vi "file - read list of lines.vi"(11 "file path":path=path "\\\\rus-one\\newdata/data/Ultrasound/Experiment/ProbeTest/Probe10/Hg1201-6-C185-550Cair-3c-83K/sweep3/9w/3366_a.dat") -> (1 "first line":string, 2 "list of lines":string[](array[string]))   [LabVIEW 2015]
uses:
  <vilib>/Utility/file.llb/Read From Spreadsheet File (string).vi
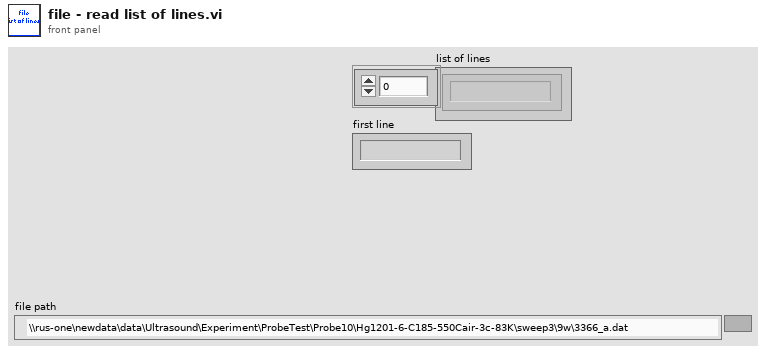
[diagram p1: front panel]
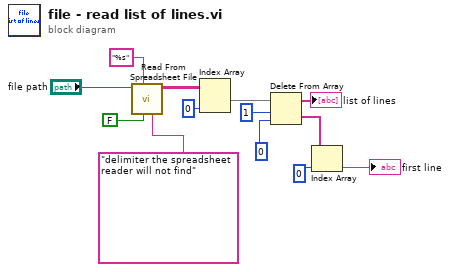
[diagram p0: block diagram]
diagram:
  n1 = call-poly <vilib>:"Read From Spreadsheet File.vi"("delimiter (\\t)"="delimiter the spreadsheet reader will not find" ("delimiter (\\t)"), "transpose (no:F)"=FALSE ("append to file? (new file:F)"), "format (%s)"="%s", "file path (dialog if empty)"="file path") -> ("all rows"=w11:string[][])  [unwired: 3 in, 4 out]
  n2 = Index Array(array=w11, index (col)=0 ("disabled index (col)")) -> (element=w9:string[])  [unwired: 1 in]
  n3 = Delete From Array(array=w9, length=1, index=0) -> (deleted portion=w4:string[], array with subset deleted=→"list of lines":string[])
  n4 = Index Array(array=w4, index=0 ("disabled index (col)")) -> (element=→"first line":string)
